vi "SW_Load_raw_data_from_TDMS.vi"(8 "error in (no error)":errorcluster, 10 "Defragment TDMS? (F)":bool, 11 "TDMS track ref. in":path) -> (0 "error out":errorcluster, 1 "SW timestamp":dbl[](array[numeric]), 2 "HW ts and Frame HW time":u32[][](array[numeric]), 3 "TDMS track ref. out":refnum<k34>, 4 "TTL IO and Key":string[][](array[string]), 5 "Raw values":dbl[][](array[numeric]))   [LabVIEW 2018, in "Tracker.lvlib"]
uses:
  Tracker.lvlib
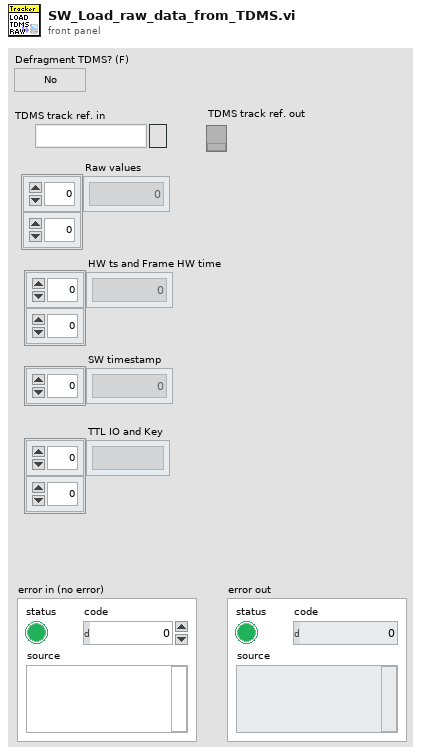
[diagram p1: front panel]
types:
  T1 = enum16{"big-endian, network order", "native, host order", "little-endian"}
  T2 = enum16{"open", "open or create", "create or replace", "create", "open (read-only)"}
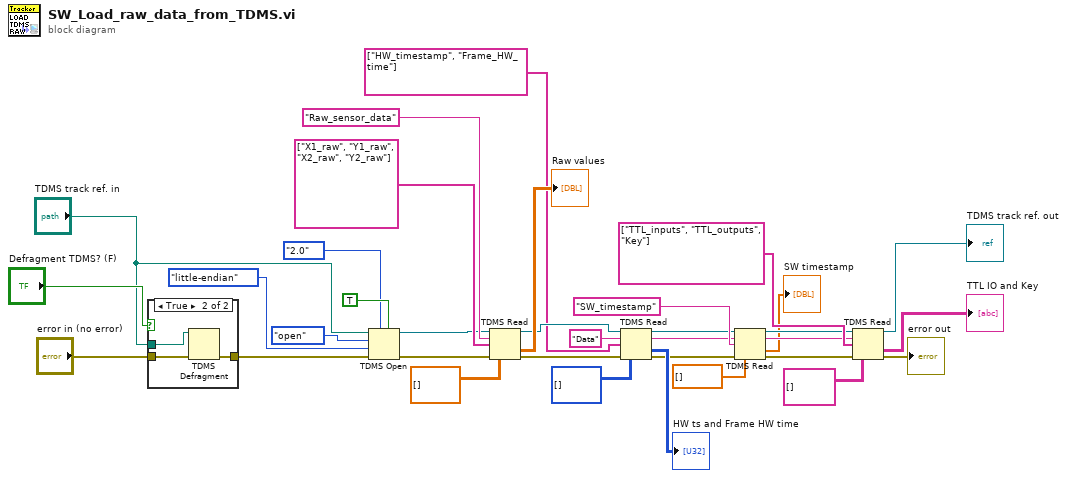
[diagram p0: block diagram]
diagram:
  n1 = case shown="True" "Defragment TDMS? (F)" {
    tunnel: "TDMS track ref. in" -> [_ w38]
    tunnel: "error in (no error)" -> [w35 w37]
    tunnel: [w35 w36] -> w5
    frame False {
    }
    frame True {
      n2 = TDMS Defragment(4:w37, 7:w38) -> (0:w36:errorcluster)
    }
  }
  n3 = TDMS Open(5:TRUE ("create index file? (T)"), 7:enum16{"1.0", "2.0"}."2.0" ("file format version (2.0)"), 8:w5, 9:T1."little-endian" ("byte order (2:little-endian)"), 10:T2."open" ("operation (0:open)"), 11:"TDMS track ref. in") -> (0:w1:errorcluster, 3:w8:refnum<k34>)  [unwired: 1 in]
  n4 = TDMS Read(0:w8, 5:"Raw_sensor_data" ("group name"), 7:string[] ["X1_raw", "Y1_raw", "X2_raw", "Y2_raw"] ("Columns Names"), 11:w1, 12:dbl[][] [] ("appended array")) -> (4:w21:refnum<k34>, 10:→"Raw values":dbl[][], 15:w33:errorcluster)  [unwired: 3 in, 3 out]
  n5 = TDMS Read(0:w21, 5:"Data" ("group name in"), 7:string[] ["HW_timestamp", "Frame_HW_time"] ("appended array"), 11:w33, 12:u32[][] [] ("appended array")) -> (4:w17:refnum<k34>, 6:w16:string, 10:→"HW ts and Frame HW time":u32[][], 15:w15:errorcluster)  [unwired: 3 in, 2 out]
  n6 = TDMS Read(0:w17, 5:w16, 7:"SW_timestamp" ("channel name(s) in (Untitled)"), 11:w15, 12:dbl[] [] ("appended array")) -> (4:w26:refnum<k34>, 6:w29:string, 10:→"SW timestamp":dbl[], 15:w27:errorcluster)  [unwired: 3 in, 2 out]
  n7 = TDMS Read(0:w26, 5:w29, 7:string[] ["TTL_inputs", "TTL_outputs", "Key"] ("channel name(s) in (Untitled)"), 11:w27, 12:string[][] [] ("appended array")) -> (4:→"TDMS track ref. out":refnum<k34>, 10:→"TTL IO and Key":string[][], 15:→"error out":errorcluster)  [unwired: 3 in, 3 out]
